vi "Drive for Distance.vi"(0 "Speed":dbl, 1 "Description":string, 5 "StartAngle":dbl=-inf, 9 "Distance (inch)":dbl, 11 "Command Info In":T1, 13 "Synchronication":enum16{"Start", "Wait"}(ring)=enum."Wait") -> (15 "Command Info Out":T1)   [LabVIEW 2017]
doc: "This VI notifies the subsystem to perform this command for the given duration, then go back to the default state. Synchronization determines whether this VI Starts the operation and returns immediately, or waits for the operation to complete. The first option is commonly used for TeleOp, and the second for Autonomous sequencing."
uses:
  <vilib>/Rock Robotics/WPI/Framework/Command Status Info.ctl
  <vilib>/Rock Robotics/WPI/Framework/Completion Status.ctl
  <vilib>/Rock Robotics/WPI/Framework/Completion Notifier.ctl
  Implementation/Drive Setpoints.ctl
  Implementation/Drive Operations.ctl
  Shared/RobotNeededPathData.ctl
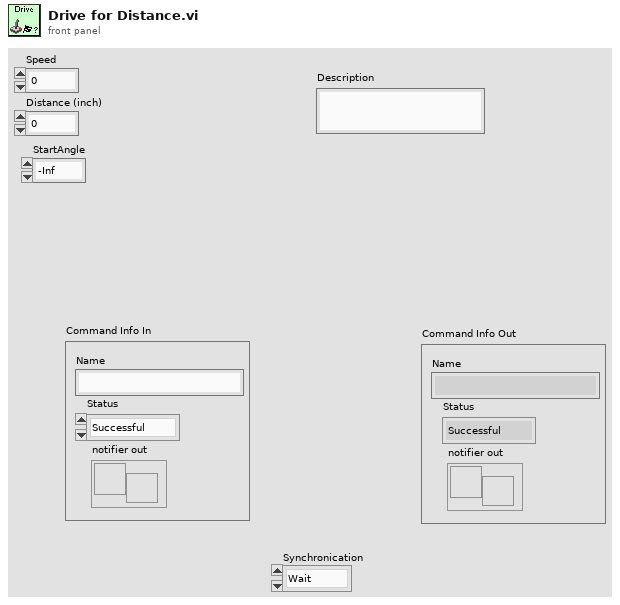
[diagram p1: front panel]
types:
  T1 = typedef "Command Status Info.ctl" = cluster{"Name":string, "Status":T2, "notifier out":T3}
  T2 = typedef "Completion Status.ctl" = enum16{"Successful", "Aborted", "Incomplete"}
  T3 = typedef "Completion Notifier.ctl" = refnum<notifier>
  T4 = typedef "Drive Setpoints.ctl" = cluster{"Operation":T5, "Left Speed":dbl, "Right Speed":dbl, "Duration":dbl, "Speed":dbl, "Start Angle":dbl, "Target Angle":dbl, "Distance (inch)":dbl, "Start Point (inch)":dbl, "RobotNeededPathData":T6, "Start Point 2":dbl}
  T5 = typedef "Drive Operations.ctl" = enum16{"Reserve", "Read Current", "Immediate", "Drive for Time", "Drive for Distance", "Turn to Angle", "Arc Turn", "Drive Path", "Drive To Cube"}
  T6 = typedef "RobotNeededPathData.ctl" = cluster{"Path":cluster{dbl, dbl}[], "MaxVel":dbl, "MaxAccel":dbl, "Backwards?":bool, "PointSpacing":dbl, "LookaheadDist":dbl, "Speed/Curve":dbl, "SlowDistanceAtEnd":dbl, "SlowSpeed":dbl}
  T7 = cluster{"Yaw":dbl, "Roll":dbl, "Pitch":dbl, "Heading":dbl, "Fused Heading":dbl}
  T8 = typedef "WPI_EncoderDevRef.ctl" = cluster{"DevStatus":errorcluster, "EncoderIndex":T9, "CounterIndex":T10, "DistancePerCount":dbl, "Decoding Type":T11}
  T9 = typedef "FPGA_EncoderIdx.ctl" = enum8{"Enc 0", "Enc 1", "Enc 2", "Enc 3", "Enc 4", "Enc 5", "Enc 6", "Enc 7", "Invalid"}
  T10 = typedef "FPGA_CounterCtrSystemIndex.ctl" = enum8{"Ctr 0", "Ctr 1", "Ctr 2", "Ctr 3", "Ctr 4", "Ctr 5", "Ctr 6", "Ctr 7", "Invalid"}
  T11 = typedef "WPI_EncoderType.ctl" = enum16{"1x", "2x", "4x"}
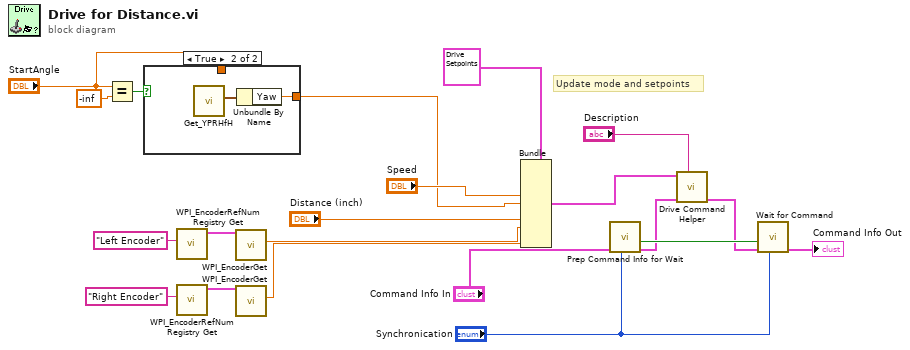
[diagram p0: block diagram]
diagram:
  # "Update mode and setpoints"
  n1 = Equal?(x="StartAngle", y=-inf) -> (x = y?=w3:bool)
  n2 = case shown="True" w3 {
    tunnel: [w22 w23] -> w1
    tunnel: "StartAngle" -> [w22 _]
    frame False {
    }
    frame True {
      n3 = call <vilib>:"Get_YPRHfH.vi"() -> ("YRPHfH"=w24:T7)  [unwired: 11 in]
      n4 = Unbundle By Name(w24) -> ("Yaw"=w23:dbl)
    }
  }
  n5 = call <vilib>:"WPI_EncoderRefNum Registry Get.vi"("refnum name"="Left Encoder") -> ("EncoderDevRef"=w9:T8)  [unwired: 9 in, 1 out]
  n6 = call <vilib>:"WPI_EncoderRefNum Registry Get.vi"("refnum name"="Right Encoder") -> ("EncoderDevRef"=w7:T8)  [unwired: 9 in, 1 out]
  n7 = call <vilib>:"WPI_EncoderGet.vi"("EncoderDevRef"=w9) -> ("Distance"=w8:dbl)  [unwired: 5 in, 5 out]
  n8 = call <vilib>:"WPI_EncoderGet.vi"("EncoderDevRef"=w7) -> ("Distance"=w5:dbl)  [unwired: 5 in, 5 out]
  n9 = Bundle(cluster=T4 {"Operation"=enum."Drive for Distance", "Left Speed"=0.0, "Right Speed"=0.0, "Duration"=0.0, "Speed"=0.0, "Start Angle"=0.0, "Target Angle"=0.0, "Distance (inch)"=0.0, "Start Point (inch)"=0.0, "RobotNeededPathData"={"Path"=[], "MaxVel"=0.0, "MaxAccel"=0.0, "Backwards?"=FALSE, "PointSpacing"=0.0, "LookaheadDist"=0.0, "Speed/Curve"=1.8, "SlowDistanceAtEnd"=12.0, "SlowSpeed"=15.0}, "Start Point 2"=0.0} ("SubSystem Data"), "Speed"="Speed", "Start Angle"=w1, "Distance (inch)"="Distance (inch)", "Start Point (inch)"=w8, "Start Point 2"=w5) -> (w14:T4)  [unwired: 6 in]
  n10 = call <vilib>:"Prep Command Info for Wait.vi"("Synchronication"="Synchronication", "Command Info"="Command Info In") -> ("Command Info"=w18:T1, "Allocated"=w19:bool)  [unwired: 8 in]
  n11 = call "Drive Command Helper.vi"("Description"="Description", "Command Info In"=w18, "SubSystem Data"=w14) -> ("Command Info Out"=w15:T1)  [unwired: 6 in, 2 out]
  n12 = call <vilib>:"Wait for Command.vi"("Synchronication"="Synchronication", "Command Info in"=w15, "Allocated"=w19) -> ("Command Info out"=→"Command Info Out":T1)  [unwired: 8 in]
